vi "Config_3457_Read.vi"(8 "error in (no error)":errorcluster) -> (0 "error out":errorcluster)   [LabVIEW 2020]
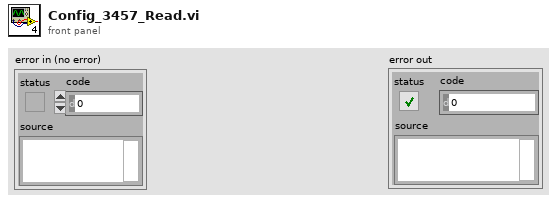
[diagram p1: front panel]
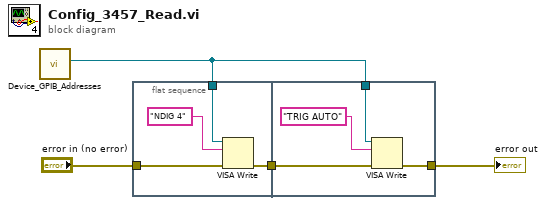
[diagram p0: block diagram]
diagram:
  n1 = call "Device_GPIB_Addresses.vi"() -> ("HP 3457A Address"=w1:refnum<visa-resource-name>)  [unwired: 9 in, 2 out]
  n2 = flat-sequence {
    tunnel: w1 -> [w7]
    tunnel: "error in (no error)" -> [w6]
    tunnel: [w5] -> w3
    tunnel: w3 -> [w11]
    tunnel: [w10] -> w2
    tunnel: w1 -> [w9]
    frame #0 {
      n3 = VISA Write(VISA resource name=w7, write buffer="NDIG 4", error in (no error)=w6) -> (error out=w5:errorcluster)  [unwired: 2 out]
    }
    frame #1 {
      n4 = VISA Write(VISA resource name=w9, write buffer="TRIG AUTO", error in (no error)=w11) -> (error out=w10:errorcluster)  [unwired: 2 out]
    }
  }
  "error out" <- w2
